vi "cntlRefs.vi"(11 "cntlRefs":T1) -> (3 "cntlRefs":T1)   [LabVIEW 2018]
doc: "This VI sets and gets certain Control References in the main VI."
uses:
  TypeDefs/cntlRefs.ctl
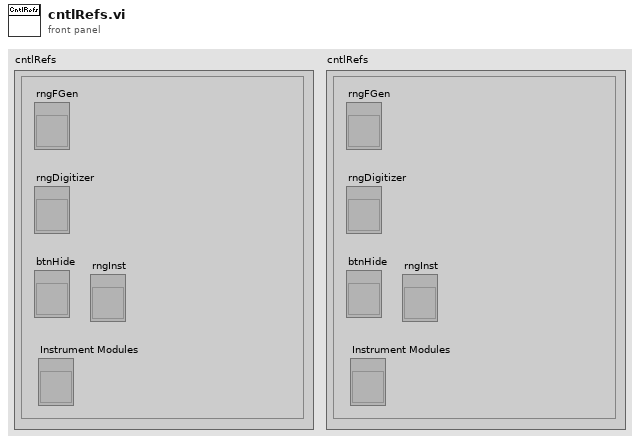
[diagram p1: front panel]
types:
  T1 = typedef "cntlRefs.ctl" = cluster{"rngFGen":refnum<vi>, "rngDigitizer":refnum<vi>, "btnHide":refnum<vi>, "rngInst":refnum<vi>, "Instrument Modules":refnum<vi>}
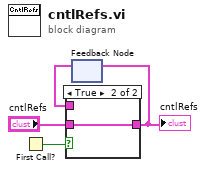
[diagram p0: block diagram]
diagram:
  n1 = First Call?() -> (First Call?: T/F=w4:bool)
  n2 = feedback #1() -> (w3:T1)  [unwired: 1 in]
  n3 = case shown="True" w4 {
    tunnel: "cntlRefs" -> [_ w6]
    tunnel: [w5 w6] -> w1
    tunnel: w3 -> [w5 _]
    frame False {
    }
    frame True {
    }
  }
  "cntlRefs" <- w1
  n4 = feedback-in #1(w1) -> ()
